vi "UUT Error Dialog.vi"(10 "Error Message":string) -> ()   [LabVIEW 2010]
uses:
  _TypeDefs/OK Button_TouchScreen.ctl
panel:
  out "Error Message Indicator":string
  out "Message":string
  in  "OK":T1
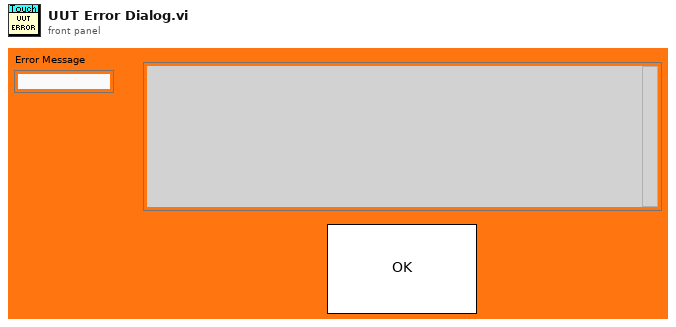
[diagram p1: front panel]
types:
  T1 = typedef "OK Button_TouchScreen.ctl" = bool
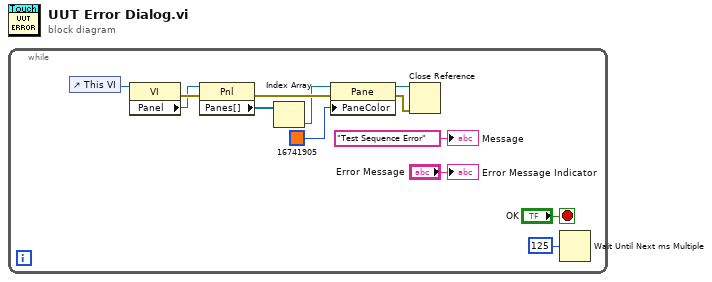
[diagram p0: block diagram]
diagram:
  n1 = while {
    stop <- "OK" stop-if-true
    n2 = control-ref of="This VI"() -> (w3:refnum<vi>)
    n3 = property class="VI"(reference=w3) -> (error out=w10:errorcluster, "Panel"=w9:refnum<vi>)  [unwired: 1 in, 1 out]
    n4 = property class="Pnl"(reference=w9, error in=w10) -> (error out=w8:errorcluster, "Panes[]"=w11:refnum<vi>[])  [unwired: 1 out]
    n5 = Index Array(array=w11) -> (element=w7:refnum<vi>)  [unwired: 1 in]
    n6 = property class="Pane"(reference=w7, error in=w8, "PaneColor"=u32 16741905) -> (reference out=w6:refnum<vi>, error out=w5:errorcluster)
    n7 = Close Reference(reference=w6, error in (no error)=w5) -> ()  [unwired: 1 out]
    n8 = Wait Until Next ms Multiple(millisecond multiple=u32 125) -> ()  [unwired: 1 out]
    "Message" <- "Test Sequence Error" ("Message")
    "Error Message Indicator" <- "Error Message"
  }
